vi "ReadRunState.vi"(8 "error in (no error)":errorcluster, 11 "AirCondition in":refnum<class "AirCondition.lvclass">) -> (0 "error out":errorcluster, 2 "RunState":bool, 3 "AirCondition out":refnum<class "AirCondition.lvclass">)   [LabVIEW 2013, in "AirCondition.lvclass"]
uses:
  AirCondition.lvclass
  AirCondition.lvclass/AirCondition.ctl
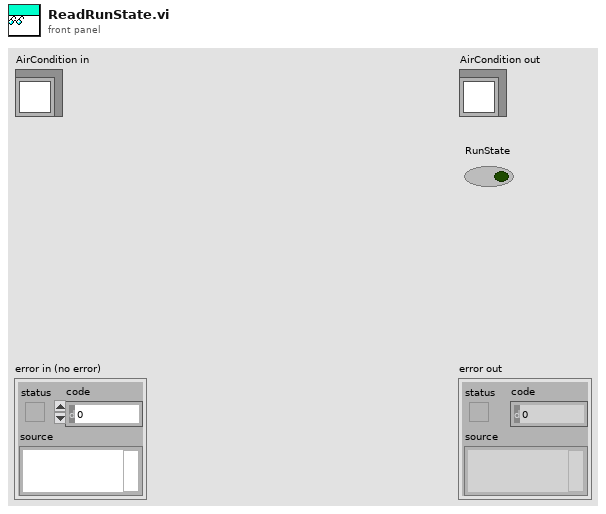
[diagram p1: front panel]
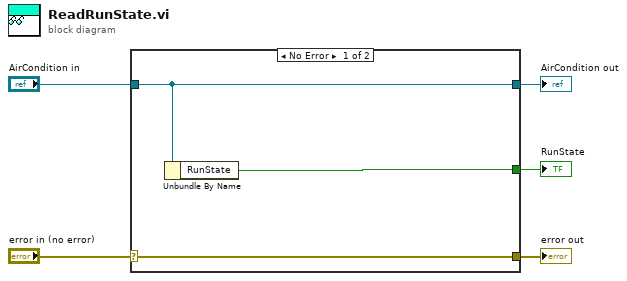
[diagram p0: block diagram]
diagram:
  n1 = case shown="No Error" "error in (no error)" {
    selector: "error in (no error)" -> [w8 w9]
    tunnel: [w8 w9] -> w4
    tunnel: [w7 w10] -> w2
    tunnel: "AirCondition in" -> [w7 w10]
    tunnel: [w6 _] -> w1
    frame No Error {
      n2 = Unbundle By Name(w7) -> ("RunState"=w6:bool)
    }
    frame Error {
    }
  }
  "error out" <- w4
  "AirCondition out" <- w2
  "RunState" <- w1
